vi "Write Pixel.vi"(8 "error in (no error)":errorcluster, 9 "Color":u32(colorbox), 10 "indices":T1, 11 "Picture in":refnum<class "Picture.lvclass">) -> (0 "error out":errorcluster, 3 "Picture out":refnum<class "Picture.lvclass">)   [LabVIEW 2018, in "Picture.lvclass"]
uses:
  Picture.lvclass
  Coords.ctl
  Picture.lvclass/Picture.ctl
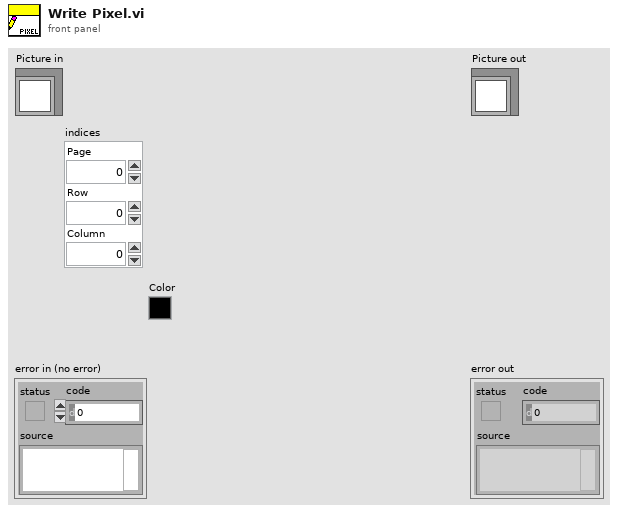
[diagram p1: front panel]
types:
  T1 = typedef "Coords.ctl" = cluster{"Page":i32, "Row":i32, "Column":i32}
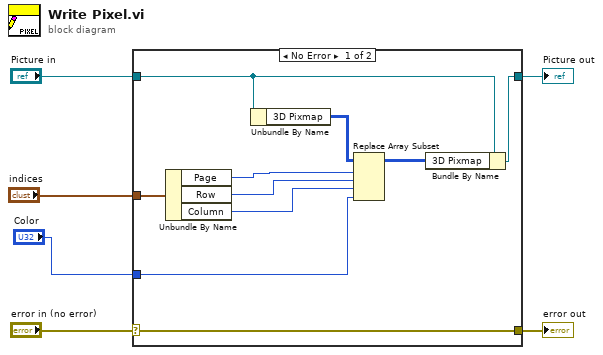
[diagram p0: block diagram]
diagram:
  n1 = case shown="No Error" "error in (no error)" {
    selector: "error in (no error)" -> [w16 w17]
    tunnel: [w16 w17] -> w5
    tunnel: [w15 w18] -> w3
    tunnel: "Picture in" -> [w8 w18]
    tunnel: "Color" -> [w12 _]
    tunnel: "indices" -> [w11 _]
    frame No Error {
      n2 = Unbundle By Name(w11) -> ("Page"=w7:i32, "Row"=w10:i32, "Column"=w9:i32)
      n3 = Unbundle By Name(w8) -> ("3D Pixmap"=w13:u32[][][])
      n4 = Replace Array Subset(array=w13, new element=w12, index (dim 0)=w7, index (dim 1)=w10, index (dim 2)=w9) -> (w14:u32[][][])
      n5 = Bundle By Name(cluster=w8, "3D Pixmap"=w14) -> (w15:refnum<class "Picture.lvclass">)
    }
    frame Error {
    }
  }
  "error out" <- w5
  "Picture out" <- w3
